vi "Unflatten String 1D.vi"(11 "Tag value":string) -> (3 "String Array 1D":string[](array[string]))   [LabVIEW 2020, in "NI_VIAn_XML Parsing.lvlib"]
uses:
  <vilib>/addons/analyzer/XML Parsing/NI_VIAn_XML Parsing.lvlib
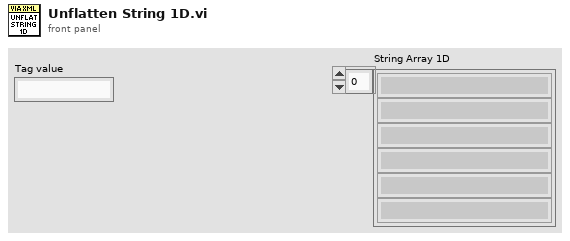
[diagram p1: front panel]
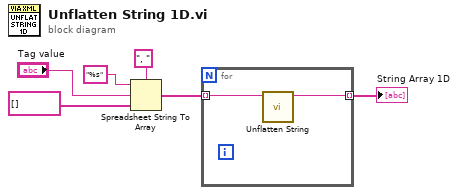
[diagram p0: block diagram]
diagram:
  n1 = Spreadsheet String To Array(delimiter (Tab)=", ", format string="%s", spreadsheet string="Tag value", array type (2D Dbl)=string[] []) -> (array=w2:string[])
  n2 = for {
    tunnel: w2 -> [w8] mode=indexing
    tunnel: [w7] -> w1 mode=indexing
    n3 = call <vilib>:"Unflatten String.vi"("Tag value"=w8) -> ("String"=w7:string)  [unwired: 10 in]
  }
  "String Array 1D" <- w1
